vi "Read STATUS cluster.vi"(8 "error in (no error)":errorcluster, 11 "PublisherGS in":refnum<class "PublisherGS.lvclass">) -> (0 "error out":errorcluster, 2 "STATUS cluster":T1, 3 "PublisherGS out":refnum<class "PublisherGS.lvclass">)   [LabVIEW 2018, in "PublisherGS.lvclass"]
uses:
  PublisherGS.lvclass
  PublisherGS.lvclass/PublisherGS.ctl
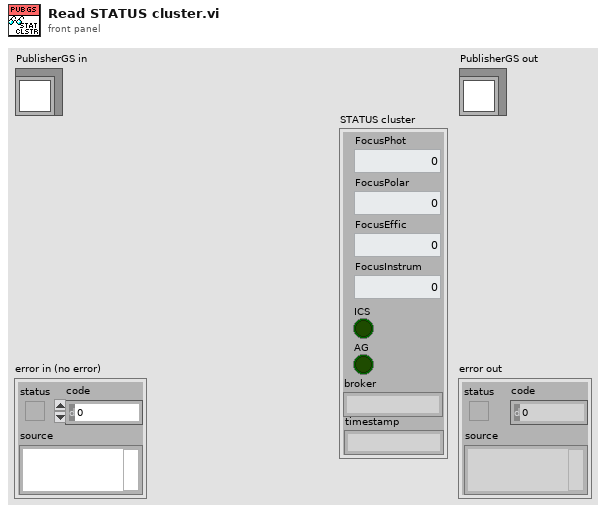
[diagram p1: front panel]
types:
  T1 = cluster{"FocusPhot":dbl, "FocusPolar":dbl, "FocusEffic":dbl, "FocusInstrum":dbl, "ICS":bool, "AG":bool, "broker":string, "timestamp":string}
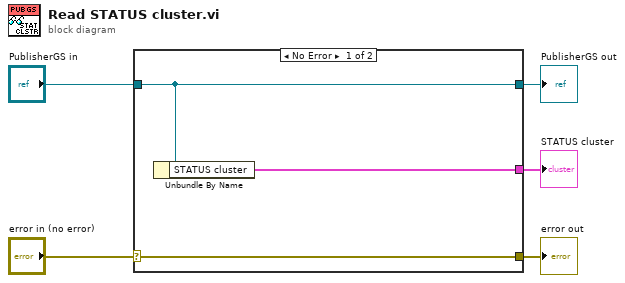
[diagram p0: block diagram]
diagram:
  n1 = case shown="No Error" "error in (no error)" {
    selector: "error in (no error)" -> [w8 w9]
    tunnel: [w8 w9] -> w4
    tunnel: [w7 w10] -> w2
    tunnel: "PublisherGS in" -> [w7 w10]
    tunnel: [w6 _] -> w1
    frame No Error {
      n2 = Unbundle By Name(w7) -> ("STATUS cluster"=w6:T1)
    }
    frame Error {
    }
  }
  "error out" <- w4
  "PublisherGS out" <- w2
  "STATUS cluster" <- w1
